vi "Close SV.vi"(8 "error in (no error)":errorcluster, 11 "AEgIS Shared Variables in":refnum<class "Circus Shared Variables.lvclass">) -> (0 "error out":errorcluster, 2 "SV":refnum<k21>, 3 "AEgIS Shared Variables out":refnum<class "Circus Shared Variables.lvclass">)   [LabVIEW 2026, in "TALOS.lvlib" / "Classes.lvlib" / "Circus Shared Variables.lvclass"]
doc: "Use this VI to close the connection to the SV. The real SV path is given as output."
uses:
  Circus Shared Variables.lvclass
  Circus Shared Variables.lvclass/Circus Shared Variables.ctl
  Ancestor/Ancestor/Ancestor.lvclass/Ancestor.ctl
  Support VIs/Generate Error.vi
  FGV/Error Memory/Get Error Description.vi
  Support VIs/Get PC name.vi
  Ancestor/Ancestor/Read ID.vi
  Support VIs/Get Class Name.vi
  <vilib>/Utility/error.llb/Clear Errors.vi
  FGV/Error Memory/Error Memory Core.vi
  <vilib>/AdvancedString/Delimited String to 1D String Array.vi
  <vilib>/AdvancedString/Delimited String to 1D String Array (string).vi
  Support VIs/Circus Root Path.vi
  FGV/Error Memory/Error Crt Lvl checker.vi
  FGV/Error Memory/Error Memory Core.vi/40c8088d-b597-4017-91af-faa98e00292e.vi
  FGV/Error Memory/Error Memory Core.vi/d4a3ab98-063c-4e44-b43d-fbdcfe6c2be2.vi
  Support VIs/Global Memory.vi
  <vilib>/Utility/LVClass/Get LV Class Name.vi
  Support VIs/Is in Packed Library.vi
  Support VIs/TALOS Root path.vi
  Support VIs/Read CSV worksheet.vi
  Support VIs/Global Constants.vi
  <vilib>/Utility/error.llb/General Error Handler.vi
  Support VIs/Error Log.vi
  Ancestor/Ancestor/Ancestor.lvclass
  <vilib>/Comparison/Equal/Equal Functor/Equal Functor.lvclass
  TALOS.lvlib
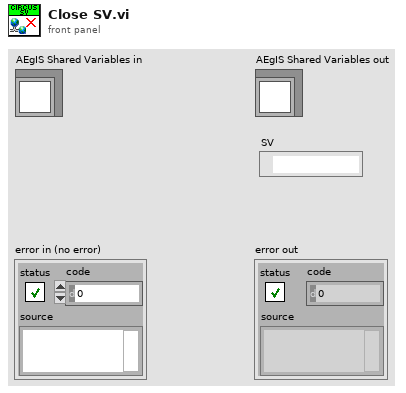
[diagram p1: front panel]
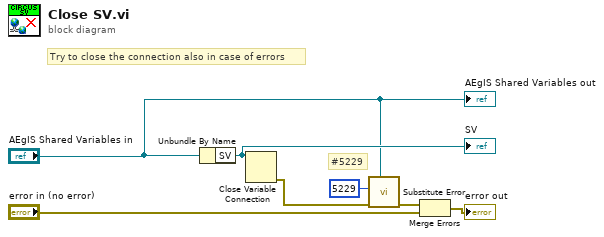
[diagram p0: block diagram]
diagram:
  # "#5229"
  # "Try to close the connection also in case of errors"
  n1 = Unbundle By Name("AEgIS Shared Variables in") -> ("SV"=w7:refnum<k21>)
  "SV" <- w7
  n2 = Close Variable Connection(11:w7) -> (0:w4:errorcluster)  [unwired: 1 in]
  n3 = call "Substitute Error.vi"("LabVIEW Object"="AEgIS Shared Variables in", "error in (no error)"=w4, "Error Code"=5229) -> ("error out"=w3:errorcluster)  [unwired: 8 in]
  n4 = Merge Errors(w3, "error in (no error)") -> (→"error out":errorcluster)
  "AEgIS Shared Variables out" <- "AEgIS Shared Variables in"
